vi "Instance.vi"(8 "error in (no error)":errorcluster) -> (0 "error out":errorcluster, 3 "Manager out":refnum<class "Manager.lvclass">)   [LabVIEW 2020, in "Parallel Block.lvlib" / "Manager.lvclass"]
uses:
  Manager.lvclass
  Manager.lvclass/Manager.ctl
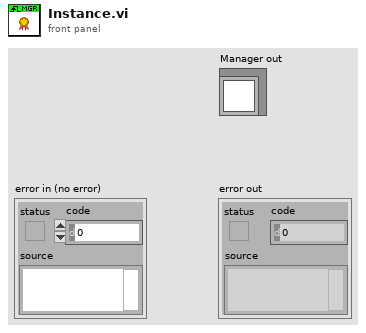
[diagram p1: front panel]
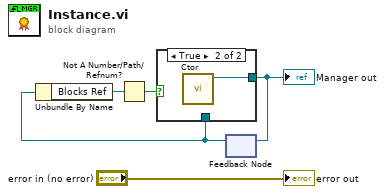
[diagram p0: block diagram]
diagram:
  n1 = feedback #1() -> (w3:refnum<class "Manager.lvclass">)  [unwired: 1 in]
  n2 = Unbundle By Name(w3) -> ("Blocks Ref"=w2:refnum<data-value>)
  n3 = Not A Number/Path/Refnum?(number/path/refnum=w2) -> (NaN/Path/Refnum?=w1:bool)
  n4 = case shown="True" w1 {
    tunnel: [w6 w7] -> w4
    tunnel: w3 -> [w6 _]
    frame False {
    }
    frame True {
      n5 = call "Ctor.vi"() -> ("Manager out"=w7:refnum<class "Manager.lvclass">)  [unwired: 10 in, 1 out]
    }
  }
  "Manager out" <- w4
  n6 = feedback-in #1(w4) -> ()
  "error out" <- "error in (no error)"
